vi "school class schedule planning simulation.vi"() -> ()   [LabVIEW 2009]
panel:
  in  "periods per day":i32
  out "progress":i32(slide) scale=0.01..95.0
  out "Waveform Graph":dbl[][](graph)
  in  "min class size":i32=5
  in  "max class size":i32=100
  out "number of class courses":i32
  in  "classes per student":i32=6
  in  "number of students":i32(slide)=100 scale=20.0..1000.0
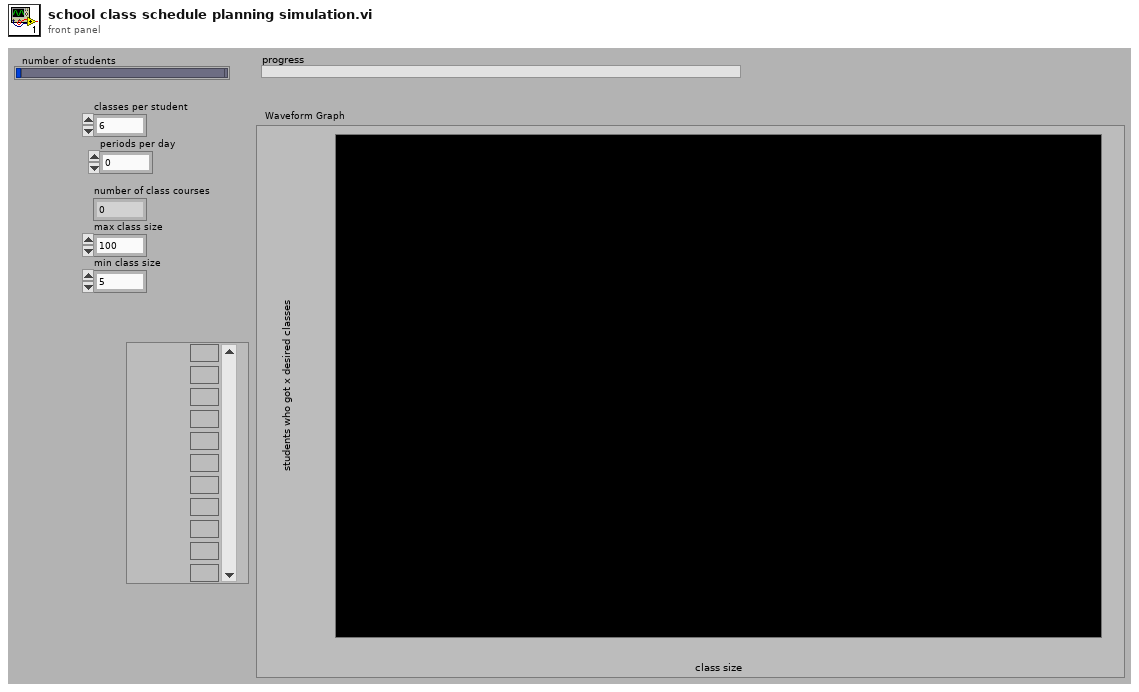
[diagram p1: front panel]
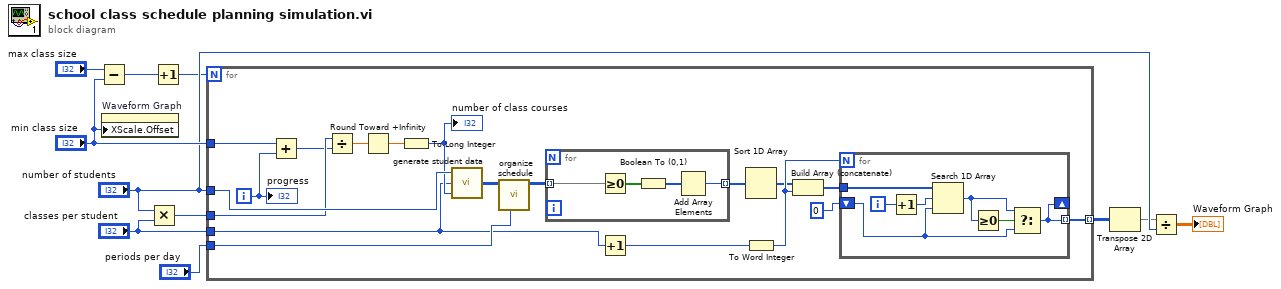
[diagram p0: block diagram]
diagram:
  n1 = Subtract(x="max class size", y="min class size") -> (x-y=w1:i32)
  n2 = property on="Waveform Graph" class="WFGraph (strict)"("XScale.Offset"="min class size") -> ()  [unwired: 2 in, 2 out]
  n3 = Multiply(x="number of students", y="classes per student") -> (x*y=w2:i32)
  n4 = Increment(x=w1) -> (x+1=w4:i32)
  n5 = for {
    N: w4 -> [_]
    tunnel: "classes per student" -> [w13]
    tunnel: "number of students" -> [w29]
    tunnel: w2 -> [w28]
    tunnel: [w12] -> w3 mode=indexing
    tunnel: "min class size" -> [w26]
    tunnel: "periods per day" -> [w23]
    i -> [w22]
    n6 = Add(x=w26, y=w22) -> (x+y=w25:i32)
    n7 = Divide(x=w28, y=w25) -> (x/y=w27:dbl)
    n8 = Round Toward +Infinity(x=w27) -> (ceil(x): smallest int >= x=w24:dbl)
    n9 = To Long Integer(number=w24) -> (32bit integer=w21:i32)
    "number of class courses" <- w21
    n10 = call "generate student data.vi"("number of class courses"=w21, "classes per student"=w13, "number of students"=w29) -> ("Student data"=w30:i32[][])
    n11 = call "organize schedule.vi"("periods per day"=w23, "Student data"=w30) -> ("rearranged Student data"=w14:i32[][])  [unwired: 9 in]
    n12 = for {
      tunnel: w14 -> [w41] mode=indexing
      tunnel: [w38] -> w15 mode=indexing
      n13 = Greater Or Equal To 0?(x=w41) -> (x >= 0?=w40:bool[])
      n14 = Boolean To (0,1)(Boolean=w40) -> (0, 1=w39:i16[])
      n15 = Add Array Elements(numeric array=w39) -> (sum=w38:i16)
    }
    n16 = Increment(x=w13) -> (x+1=w17:i32)
    n17 = Sort 1D Array(array=w15) -> (sorted array=w16:i16[])
    n18 = To Word Integer(number=w17) -> (16bit integer=w20:i16)
    n19 = Build Array (concatenate)(w16, w20) -> (w18:i16[])
    n20 = for {
      N: w20 -> [_]
      tunnel: w18 -> [w37]
      shift-right: [w31] -> _
      shift-left: 0 ("index of element") -> [w34]
      tunnel: [w31] -> w12 mode=indexing
      i -> [w36]
      n21 = Increment(x=w36) -> (x+1=w35:i32)
      n22 = Search 1D Array(1D array=w37, element=w35, start index (0)=w34) -> (index of element=w33:i32)
      n23 = Greater Or Equal To 0?(x=w33) -> (x >= 0?=w32:bool)
      n24 = Select(t=w33, s=w32, f=w34) -> (s? t:f=w31:i32)
    }
    "progress" <- w22
  }
  n25 = Transpose 2D Array(2D array=w3) -> (transposed array=w5:i32[][])
  n26 = Divide(x=w5, y="number of students") -> (x/y=→"Waveform Graph":dbl[][])
